vi "数据时间对齐处理.vi"(9 "待对齐时间":timestamp, 10 "对齐参考时间":timestamp, 11 "已对齐时间输入":timestamp) -> (2 "数组":timestamp[](array[timestamp]), 3 "已对齐时间输出":timestamp)   [LabVIEW 2016, in "斯坦道氨氮.lvlib"]
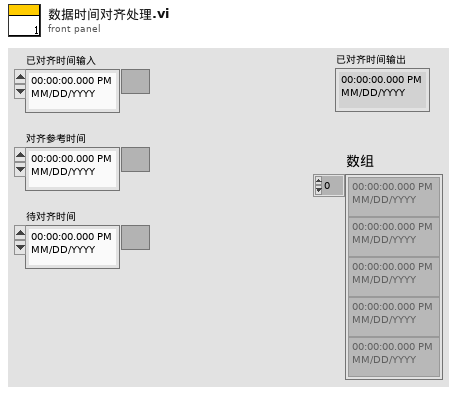
[diagram p1: front panel]
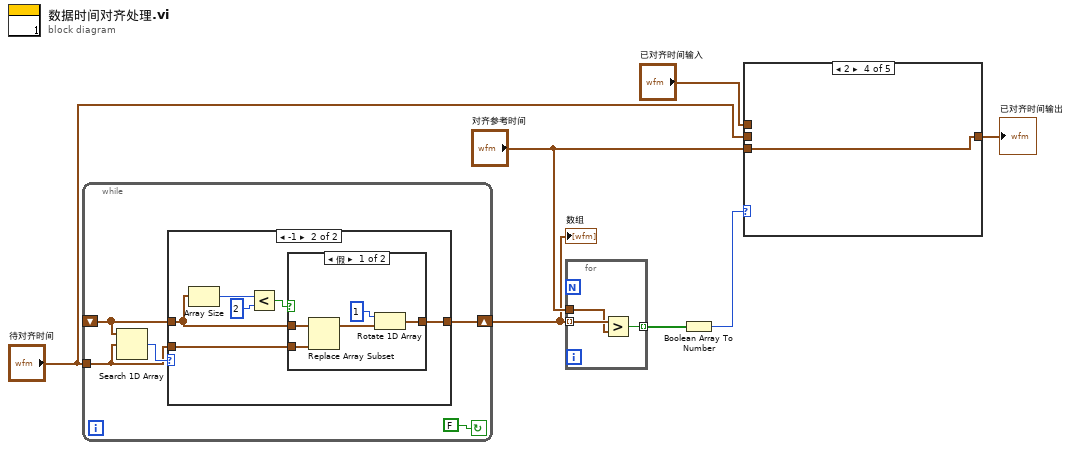
[diagram p0: block diagram]
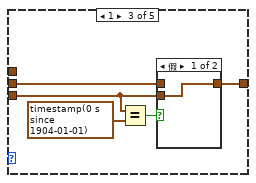
[diagram p4: hidden frame]
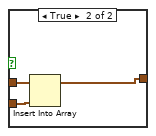
[diagram p8: hidden frame]
diagram:
  n1 = while {
    shift-right: [w9] -> w1
    shift-left: _ -> [w11]
    tunnel: "待对齐时间" -> [w10]
    stop <- FALSE continue-if-true
    n2 = Search 1D Array(1D array=w11, element=w10) -> (index of element=w12:i32)  [unwired: 1 in]
    n3 = case shown="-1" w12 {
      tunnel: w11 -> [w13 w17]
      tunnel: w10 -> [_ w19]
      tunnel: [w13 w18] -> w9
      frame 0, Default {
      }
      frame -1 {
        n4 = Array Size(array=w17) -> (size(s)=w16:i32)
        n5 = Less?(x=w16, y=2) -> (x < y?=w14:bool)
        n6 = case shown="假" w14 {
          tunnel: w19 -> [w24 w27]
          tunnel: [w20 w26] -> w18
          tunnel: w17 -> [w22 w25]
          frame False {
            n7 = Replace Array Subset(array=w22, new element=w24) -> (w21:timestamp[])  [unwired: 1 in]
            n8 = Rotate 1D Array(1:w21, 2:1 ("n")) -> (0:w20:timestamp[])
          }
          frame True {
            n9 = Insert Into Array(array=w25, new element=w27) -> (w26:timestamp[])  [unwired: 1 in]
          }
        }
      }
    }
  }
  "数组" <- w1
  n10 = for {
    tunnel: w1 -> [w30] mode=indexing
    tunnel: "对齐参考时间" -> [w29]
    tunnel: [w28] -> w2 mode=indexing
    n11 = Greater?(x=w30, y=w29) -> (0:w28:bool)
  }
  n12 = Boolean Array To Number(Boolean array=w2) -> (number=w5:u32)
  n13 = case shown="2" w5 {
    tunnel: [w31 w32 w34 w40 w41] -> w7
    tunnel: "待对齐时间" -> [w31 _ w35 _ w41]
    tunnel: "对齐参考时间" -> [_ _ w33 w40 _]
    tunnel: "已对齐时间输入" -> [_ w32 _ _ _]
    frame Default {
    }
    frame 0 {
    }
    frame 1 {
      n14 = Equal?(x=w33, y=timestamp(0 s since 1904-01-01)) -> (x = y?=w36:bool)
      n15 = case shown="假" w36 {
        tunnel: w35 -> [_ w39]
        tunnel: [w38 w39] -> w34
        tunnel: w33 -> [w38 _]
        frame False {
        }
        frame True {
        }
      }
    }
    frame 2 {
    }
    frame 3 {
    }
  }
  "已对齐时间输出" <- w7
